vi "oax_AI Config (DAQmx DSA).vi"(6 "reset devices (false)":bool, 7 "buffer size":u32=10000, 8 "error in (no error)":errorcluster, 9 "min value":dbl=-5.0 format="%0.2f", 10 "max value":dbl=5.0 format="%0.2f", 11 "DAQ Config":T1 {"pregain" format="%.2f"; "IEPE" items=["On", "Off", "None"]; "coupling" items=["DC", "AC"]; "engineering units" items=["custom..."=0, "V"=1, "A"=21, "C"=30, "pC"=31, "s"=32, "-"=29, "Pa"=2, "N"=20, "g"=3, "m/s^2"=4, "m/s"=5, "m"=6, "mm/s"=12, "mm"=13, "micron/s"=14, "micron"=15, "in/s^2"=7, "in/s"=8, "in"=9, "mil/s"=10, "mil"=11, "rad/s^2"=16, "rad/s"=17, "rad"=18, "deg/s^2"=26, "deg/s"=27, "deg"=28, "RPM"=22, "cycle/s^2"=23, "Hz"=24, "cycle"=25, "strain"=19]; "sensor sensitivity (mV/EU)" format="%.2f"; "dB reference" format="%.1e"}) -> (0 "error out":errorcluster, 3 "task out":refnum<k21>)   [LabVIEW 2017]
doc: "Reset devices and creates a DAQmx AI Voltage task, configure IEPE excitation, and input coupling."
uses:
  <vilib>/addons/Sound and Vibration/Order Analysis/Example Support/sub VIs/OAXML_DSA DAQ Config.ctl
  <vilib>/addons/_NISVFA/_Shared subVIs/Controls/svc_Engineering Units Text Ring.ctl
  <vilib>/DAQmx/create/channels.llb/DAQmx Create Channel (AI-Voltage-Basic).vi
  <resource>/objmgr/daqmx.rc
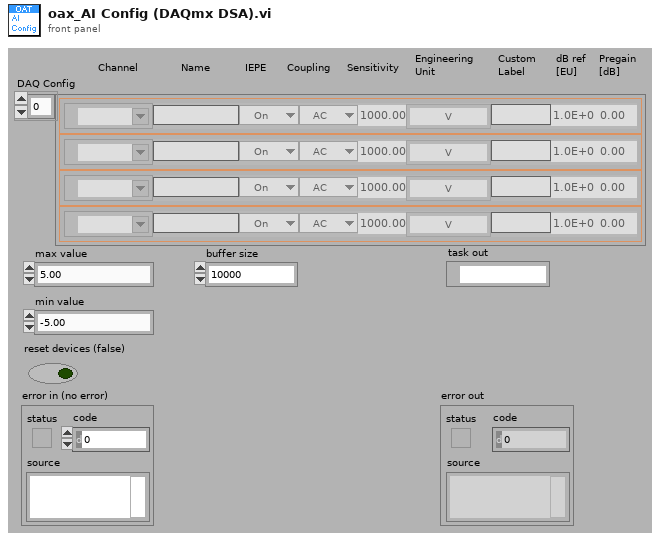
[diagram p1: front panel]
types:
  T1 = typedef "OAXML_DSA DAQ Config.ctl" = cluster{"name":string, "channel":tag, "coupling":u16, "dB reference":sgl, "sensor sensitivity (mV/EU)":dbl, "engineering units":T2, "IEPE":u16, "custom label":string, "pregain":sgl}[]
  T2 = typedef "svc_Engineering Units Text Ring.ctl" = u16
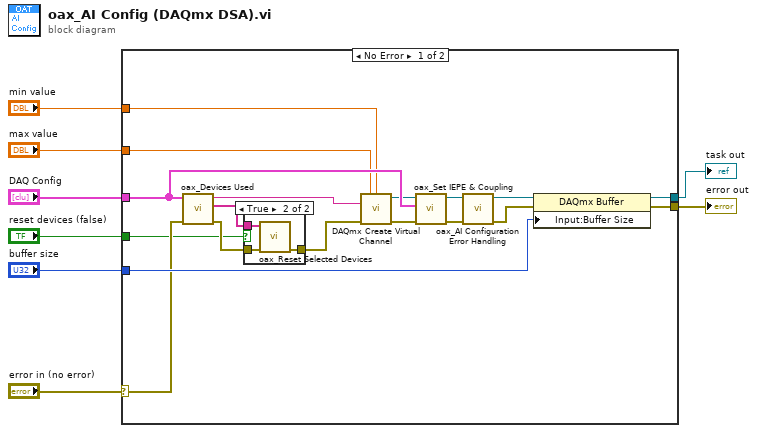
[diagram p0: block diagram]
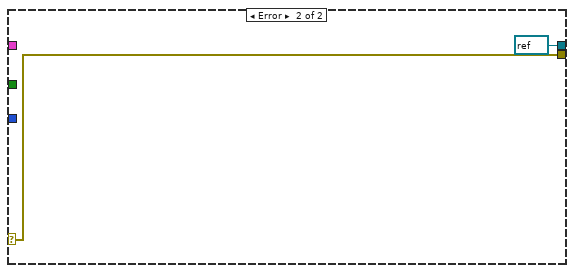
[diagram p3: hidden frame]
diagram:
  n1 = case shown="No Error" "error in (no error)" {
    selector: "error in (no error)" -> [w24 w32]
    tunnel: "DAQ Config" -> [w26 _]
    tunnel: "buffer size" -> [w25 _]
    tunnel: "max value" -> [w23 _]
    tunnel: "min value" -> [w22 _]
    tunnel: [w21 w32] -> w2
    tunnel: [w20 refnum<k21> refnum ("task out")] -> w3
    tunnel: "reset devices (false)" -> [w9 _]
    frame No Error {
      n2 = call <vilib>:"oax_Devices Used.vi"("error in"=w24, "DAQ Config"=w26) -> ("error out"=w18:errorcluster, "devices used"=w19:string[], "Channels list"=w16:string)  [unwired: 7 in]
      n3 = case shown="True" w9 {
        tunnel: w19 -> [_ w30]
        tunnel: w18 -> [w27 w29]
        tunnel: [w27 w28] -> w17
        frame False {
        }
        frame True {
          n4 = call <vilib>:"oax_Reset Selected Devices.vi"("error in"=w29, "devices to reset"=w30) -> ("error out"=w28:errorcluster)  [unwired: 9 in]
        }
      }
      n5 = call-poly <vilib>:"DAQmx Create Virtual Channel.vi"("maximum value"=w23, "minimum value"=w22, "physical channels"=w16, "error in"=w17) -> ("task out"=w15:refnum<k21>, "error out"=w14:errorcluster)  [unwired: 10 in]
      n6 = call <vilib>:"oax_Set IEPE & Coupling.vi"("error in (no error)"=w14, "DAQ Config"=w26, "task in"=w15) -> ("error out"=w13:errorcluster, "task out"=w11:refnum<k21>)  [unwired: 7 in]
      n7 = call <vilib>:"oax_AI Configuration Error Handling.vi"("error in"=w13, "task in"=w11) -> ("error out"=w12:errorcluster, "task out"=w10:refnum<k21>)  [unwired: 8 in]
      n8 = property class="DAQmx Buffer"(reference=w10, error in=w12, "Input:Buffer Size"=w25) -> (reference out=w20:refnum<k21>, error out=w21:errorcluster)
    }
    frame Error {
    }
  }
  "error out" <- w2
  "task out" <- w3
